vi "Ramp Calibration Logic.vi"() -> ()   [LabVIEW 2026]
panel:
  out "LIMIT WARNING":bool
  out "Scaled Float Output":dbl
  in  "milliseconds to wait":u32
  in  "LOOP COUNT":i32
  out "LOOP ITERATION":i32
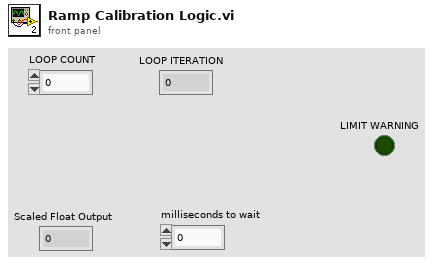
[diagram p1: front panel]
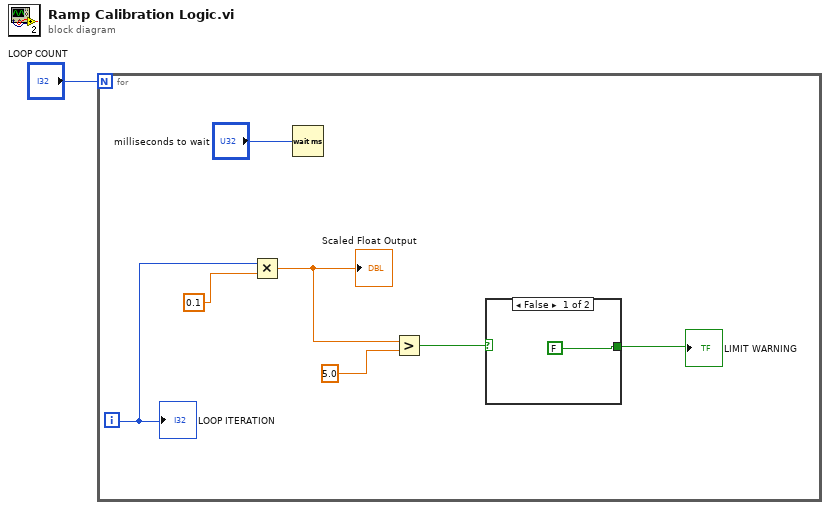
[diagram p0: block diagram]
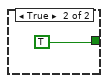
[diagram p2: hidden frame]
diagram:
  n1 = for {
    N: "LOOP COUNT" -> [_]
    i -> [w7]
    n2 = Multiply(x=w7, y=0.1) -> (x*y=w5:dbl)
    "Scaled Float Output" <- w5
    n3 = Wait (ms)(milliseconds to wait="milliseconds to wait") -> ()  [unwired: 1 out]
    n4 = Greater?(x=w5, y=5.0) -> (0:w3:bool)
    n5 = case shown="False" w3 {
      tunnel: [FALSE TRUE] -> w2
      frame False {
      }
      frame True {
      }
    }
    "LIMIT WARNING" <- w2
    "LOOP ITERATION" <- w7
  }
